vi "p1.vi"() -> ()   [LabVIEW 2023, in "d9.lvlib"]
uses:
  d9.lvlib
  AOC/AOC.lvlib
panel:
  in  "Example":string
  in  "Example":bool
  out "Answer":i64=6498
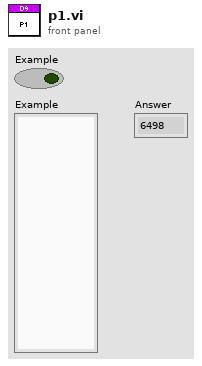
[diagram p1: front panel]
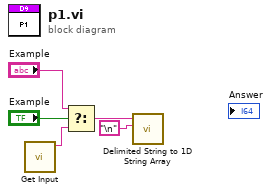
[diagram p0: block diagram]
diagram:
  n1 = call "Get Input.vi"() -> ("Input"=w1:string)  [unwired: 11 in]
  n2 = Select(t="Example", s="Example", f=w1) -> (s? t:f=w5:string)
  n3 = call <vilib>:"Delimited String to 1D String Array.vi"("delimiter"="\n", "delimited string"=w5) -> ()  [unwired: 9 in, 1 out]
